vi "Write_tcpServer_queue.vi"(8 "error in (no error)":errorcluster, 10 "tcpServer queue":refnum<queue>, 11 "tcpServer in":refnum<class "TcpServer.lvclass">) -> (0 "error out":errorcluster, 3 "tcpServer out":refnum<class "TcpServer.lvclass">)   [LabVIEW 2018, in "TcpServer.lvclass"]
doc: "Write server queue."
uses:
  TcpServer.lvclass
  TcpServer.lvclass/TcpServer.ctl
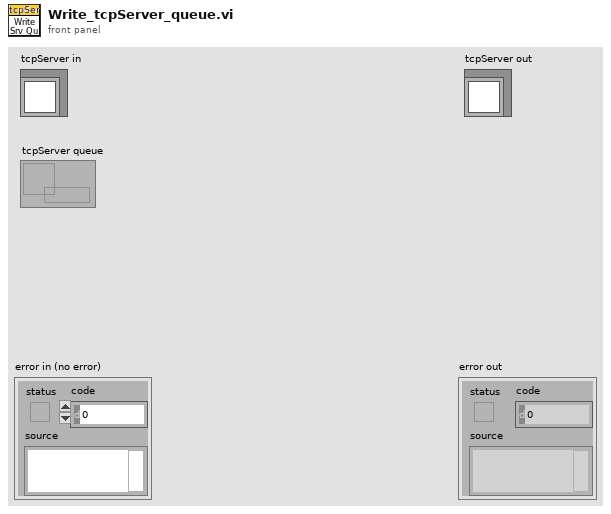
[diagram p1: front panel]
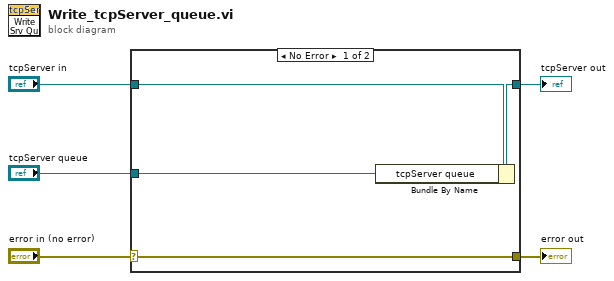
[diagram p0: block diagram]
diagram:
  n1 = case shown="No Error" "error in (no error)" {
    selector: "error in (no error)" -> [w9 w10]
    tunnel: [w9 w10] -> w4
    tunnel: [w7 w11] -> w2
    tunnel: "tcpServer in" -> [w8 w11]
    tunnel: "tcpServer queue" -> [w6 _]
    frame No Error {
      n2 = Bundle By Name(cluster=w8, "tcpServer queue"=w6) -> (w7:refnum<class "TcpServer.lvclass">)
    }
    frame Error {
    }
  }
  "error out" <- w4
  "tcpServer out" <- w2
